vi "u16_array_to_sgl_array.vi"(8 "word order":enum16{"little endian", "big endian"}(ring)=enum."big endian" caption="word order (1: big endian)", 11 "Regs_u16":u16[](array[numeric])) -> (3 "VAL_sgl":sgl[](array[numeric]) format="%.3p")   [LabVIEW 2014]
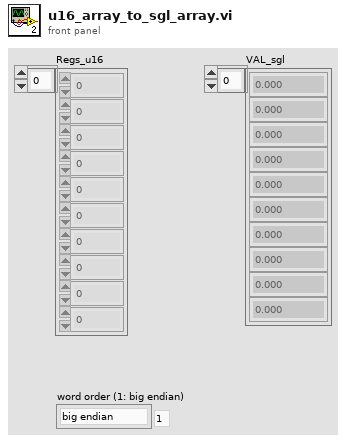
[diagram p1: front panel]
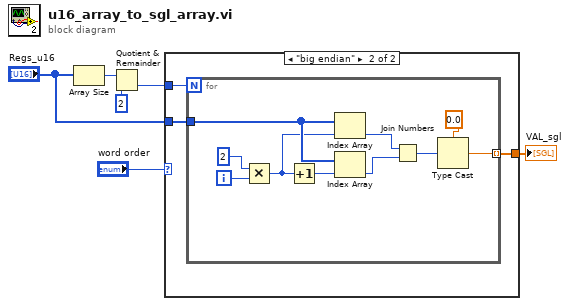
[diagram p0: block diagram]
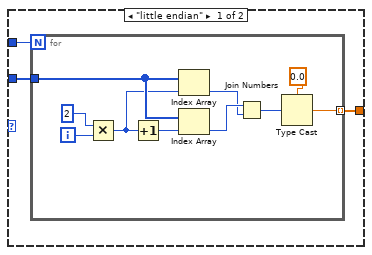
[diagram p2: hidden frame]
diagram:
  n1 = Array Size(array="Regs_u16") -> (size(s)=w6:i32)
  n2 = Quotient & Remainder(x=w6, y=2) -> (floor(x/y)=w4:i32)  [unwired: 1 out]
  n3 = case shown="\"big endian\"" "word order" {
    tunnel: w4 -> [w9 w22]
    tunnel: [w8 w21] -> w3
    tunnel: "Regs_u16" -> [w7 w20]
    frame "little endian" {
      n4 = for {
        N: w9 -> [_]
        tunnel: w7 -> [w19]
        tunnel: [w13] -> w8 mode=indexing
        i -> [w16]
        n5 = Multiply(x=2, y=w16) -> (x*y=w14:i32)
        n6 = Increment(x=w14) -> (x+1=w18:i32)
        n7 = Index Array(array=w19, index=w14) -> (element=w10:u16)
        n8 = Index Array(array=w19, index=w18) -> (element=w11:u16)
        n9 = Join Numbers(hi=w11, lo=w10) -> ((hi.lo)=w12:u32)
        n10 = Type Cast(type=sgl 0.0, x=w12) -> (*(type *) &x=w13:sgl)
      }
    }
    frame "big endian" {
      n11 = for {
        N: w22 -> [_]
        tunnel: w20 -> [w32]
        tunnel: [w26] -> w21 mode=indexing
        i -> [w29]
        n12 = Multiply(x=2, y=w29) -> (x*y=w27:i32)
        n13 = Increment(x=w27) -> (x+1=w31:i32)
        n14 = Index Array(array=w32, index=w27) -> (element=w24:u16)
        n15 = Index Array(array=w32, index=w31) -> (element=w23:u16)
        n16 = Join Numbers(hi=w24, lo=w23) -> ((hi.lo)=w25:u32)
        n17 = Type Cast(type=sgl 0.0, x=w25) -> (*(type *) &x=w26:sgl)
      }
    }
  }
  "VAL_sgl" <- w3
